vi "DC_Link_v2.vi"(8 "error in":errorcluster, 9 "# of Channels In":enum16{"1", "2"}(ring), 10 "Write Channels":string="NI9264/ao2", 11 "Read Task":string="BONTS_DC-Link_Feedback") -> (0 "error out":errorcluster, 3 "DC Gain":dbl[](array[numeric]))   [LabVIEW 2021]
uses:
  <vilib>/DAQmx/write.llb/DAQmx Write (Analog 1D Wfm NChan NSamp).vi
  <vilib>/DAQmx/read.llb/DAQmx Read (Analog 1D Wfm NChan NSamp).vi
  <vilib>/DAQmx/create/channels.llb/DAQmx Create Channel (AO-Voltage-Basic).vi
  <vilib>/DAQmx/configure/timing.llb/DAQmx Timing (Sample Clock).vi
  <vilib>/DAQmx/miscellaneous.llb/DAQmx Fill In Error Info.vi
  <vilib>/measure/madcrms.llb/Basic Averaged DC-RMS for N Chan.vi
  <resource>/objmgr/daqmx.rc
  <vilib>/measure/NI_MABase.lvlib
  <vilib>/measure/NI_MAPro.lvlib
panel:
  out "Output Signal":waveform(dbl)[](graph)
  out "Input Signal":waveform(dbl)[](graph)
  in  "Number of Samples 2":i32=1000
  in  "Sample Rate 2":dbl=1000.0
  in  "Signal 1 (5V)":tag="OnboardClock"
  out "Actual Sample Rate 2":dbl=1000.0 format="%0.2f"
  # "This test will input inverse waveforms into the DC Link -/+"
  # "And capture the DC Link Voltage, as well as the Overvoltage Fault"
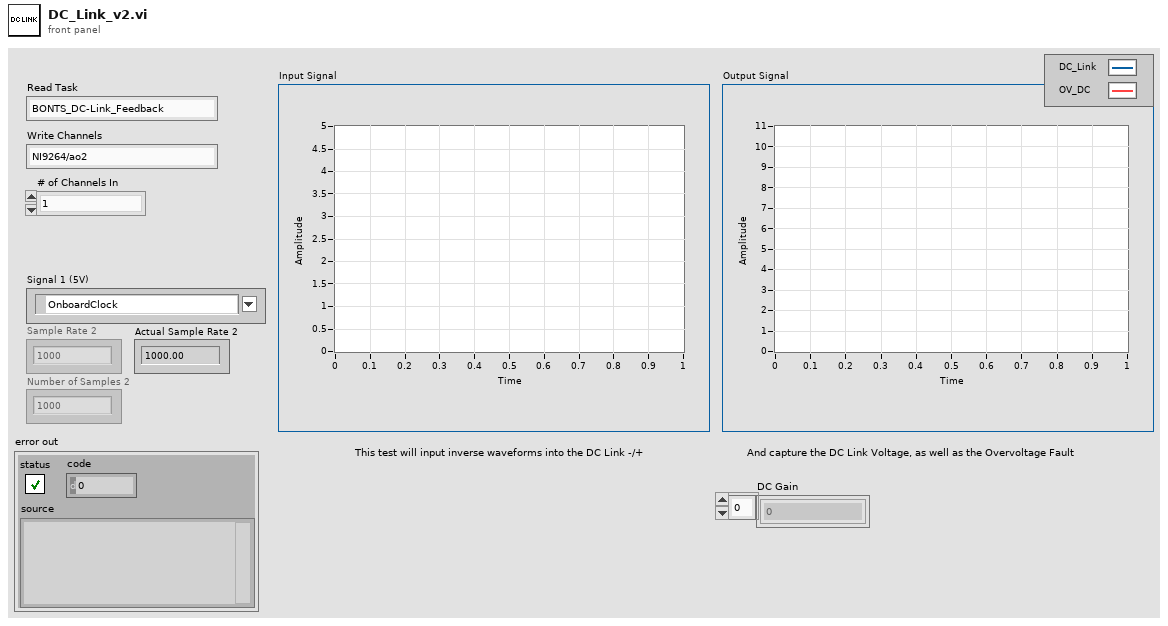
[diagram p1: front panel]
types:
  T1 = cluster{"Waveform Type":u16, "Amplitude":dbl, "Frequency":dbl}[]
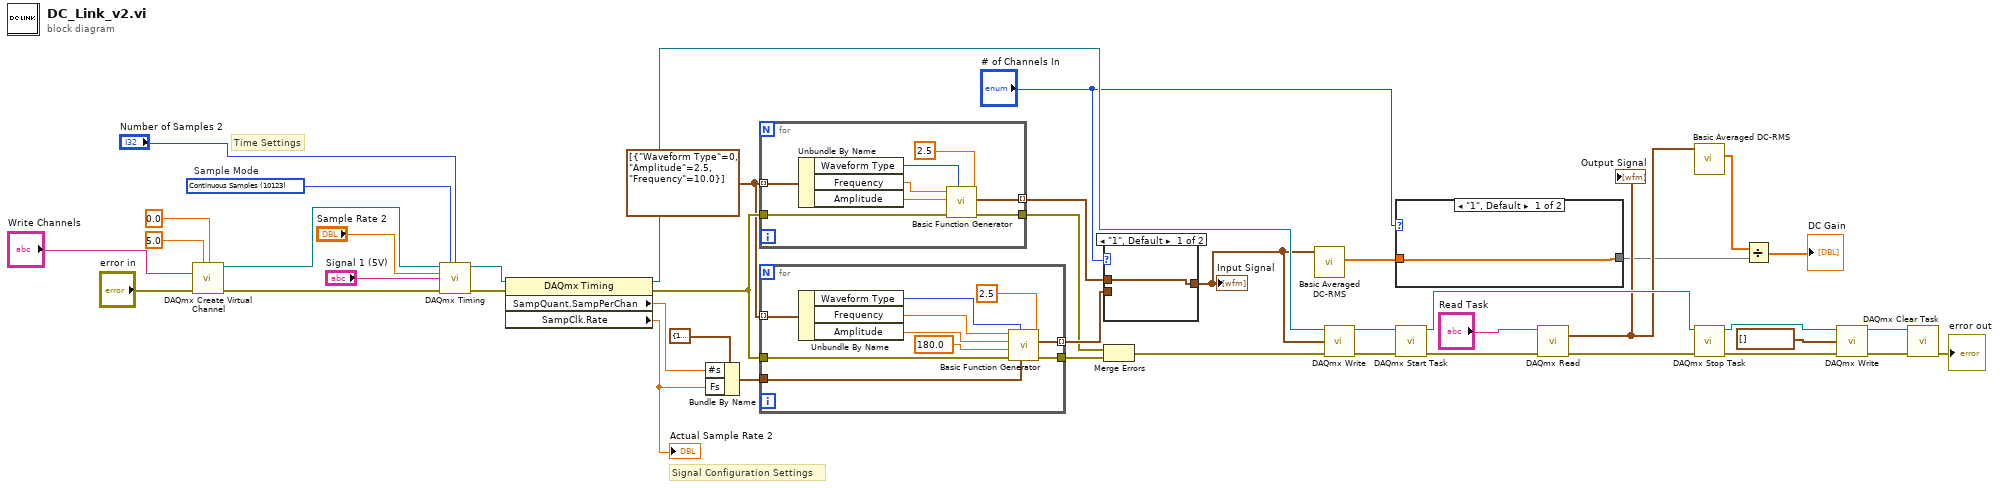
[diagram p0: block diagram]
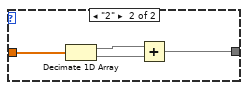
[diagram p2: hidden frame]
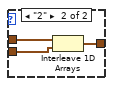
[diagram p3: hidden frame]
diagram:
  w17 = T1 [{"Waveform Type"=0, "Amplitude"=2.5, "Frequency"=10.0}] ("Signal Input")
  w34 = 10123 items=["Finite Samples"=10178, "Continuous Samples"=10123, "Hardware Timed Single Point"=12522]  # Sample Mode
  # "Time Settings"
  # "Signal Configuration Settings"
  n1 = call-poly <vilib>:"DAQmx Create Virtual Channel.vi"("maximum value"=5.0, "minimum value"=0.0, "physical channels"="Write Channels", "error in"="error in") -> ("task out"=w4:refnum<k21>, "error out"=w33:errorcluster)  [unwired: 10 in]
  n2 = call-poly <vilib>:"DAQmx Timing.vi"("task/channels in"=w4, "sample mode"=w34, "samples per channel"="Number of Samples 2", "rate"="Sample Rate 2", "source"="Signal 1 (5V)", "error in"=w33) -> ("task out"=w36:refnum<k21>, "error out"=w35:errorcluster)  [unwired: 8 in]
  n3 = property class="DAQmx Timing"(reference=w36, error in=w35) -> (reference out=w43:refnum<k21>, error out=w22:errorcluster, "SampQuant.SampPerChan"=w28:dbl, "SampClk.Rate"=w27:dbl)
  "Actual Sample Rate 2" <- w27
  n4 = Bundle By Name(cluster=cluster{"Fs":dbl, "#s":dbl} {"Fs"=1000.0, "#s"=1000.0} ("sampling info"), "#s"=w28, "Fs"=w27) -> (w23:cluster{"Fs":dbl, "#s":dbl})
  n5 = for {
    tunnel: [w51] -> w20
    tunnel: w17 -> [w50] mode=indexing
    tunnel: [w46] -> w6 mode=indexing
    tunnel: w22 -> [w45]
    n6 = Unbundle By Name(w50) -> ("Waveform Type"=w49:u16, "Frequency"=w48:dbl, "Amplitude"=w47:dbl)
    n7 = call <vilib>:"Basic Function Generator.vi"("offset"=2.5, "signal type"=w49, "error in (no error)"=w45, "amplitude"=w47, "frequency"=w48) -> ("error out"=w51:errorcluster, "signal out"=w46:waveform(dbl))  [unwired: 4 in, 1 out]
  }
  n8 = for {
    tunnel: w22 -> [w54]
    tunnel: w23 -> [w61]
    tunnel: [w60] -> w19
    tunnel: w17 -> [w59] mode=indexing
    tunnel: [w55] -> w42 mode=indexing
    n9 = Unbundle By Name(w59) -> ("Waveform Type"=w58:u16, "Frequency"=w57:dbl, "Amplitude"=w56:dbl)
    n10 = call <vilib>:"Basic Function Generator.vi"("offset"=2.5, "sampling info"=w61, "signal type"=w58, "error in (no error)"=w54, "phase"=180.0, "amplitude"=w56, "frequency"=w57) -> ("error out"=w60:errorcluster, "signal out"=w55:waveform(dbl))  [unwired: 2 in, 1 out]
  }
  n11 = case shown="\"1\", Default" "# of Channels In" {
    tunnel: w42 -> [_ w63]
    tunnel: [w62 w65] -> w5
    tunnel: w6 -> [w62 w64]
    frame "1", Default {
    }
    frame "2" {
      n12 = Interleave 1D Arrays(w64, w63) -> (w65:waveform(dbl)[])
    }
  }
  "Input Signal" <- w5
  n13 = Merge Errors(w20, w19) -> (w18:errorcluster)
  n14 = call-poly <vilib>:"Basic Averaged DC-RMS.vi"("signals in"=w5) -> ("RMS values"=w3:dbl[])  [unwired: 7 in, 3 out]
  n15 = call-poly <vilib>:"DAQmx Write.vi"("task/channels in"=w43, "data"=w5, "error in"=w18) -> ("task out"=w41:refnum<k21>, "error out"=w40:errorcluster)  [unwired: 10 in, 1 out]
  n16 = case shown="\"1\", Default" "# of Channels In" {
    tunnel: w3 -> [w66 w70]
    tunnel: [w66 w69] -> w2
    frame "1", Default {
    }
    frame "2" {
      n17 = Decimate 1D Array(w70) -> (w68:dbl[], w67:dbl[])
      n18 = Add(x=w68, y=w67) -> (x+y=w69:dbl[])
    }
  }
  n19 = call <vilib>:"DAQmx Start Task.vi"("task/channels in"=w41, "error in"=w40) -> ("task out"=w38:refnum<k21>, "error out"=w39:errorcluster)  [unwired: 12 in]
  n20 = call-poly <vilib>:"DAQmx Read.vi"("task/channels in"="Read Task", "error in"=w39) -> ("data"=w15:waveform(dbl)[], "error out"=w37:errorcluster)  [unwired: 11 in, 1 out]
  "Output Signal" <- w15
  n21 = call-poly <vilib>:"Basic Averaged DC-RMS.vi"("signals in"=w15) -> ("RMS values"=w14:dbl[])  [unwired: 7 in, 3 out]
  n22 = call <vilib>:"DAQmx Stop Task.vi"("task/channels in"=w38, "error in"=w37) -> ("task out"=w12:refnum<k21>, "error out"=w8:errorcluster)  [unwired: 12 in]
  n23 = Divide(x=w14, y=w2) -> (x/y=→"DC Gain":dbl[])
  n24 = call-poly <vilib>:"DAQmx Write.vi"("task/channels in"=w12, "data"=waveform(dbl)[] [], "error in"=w8) -> ("task out"=w11:refnum<k21>, "error out"=w9:errorcluster)  [unwired: 10 in, 1 out]
  n25 = call <vilib>:"DAQmx Clear Task.vi"("task in"=w11, "error in"=w9) -> ("error out"=→"error out":errorcluster)  [unwired: 13 in]
